vi "Finalize.vi"(3 "erreur in":errorcluster caption="eerror in", 5 "ref in":refnum<k7>) -> (0 "error out":errorcluster)   [LabVIEW 2010]
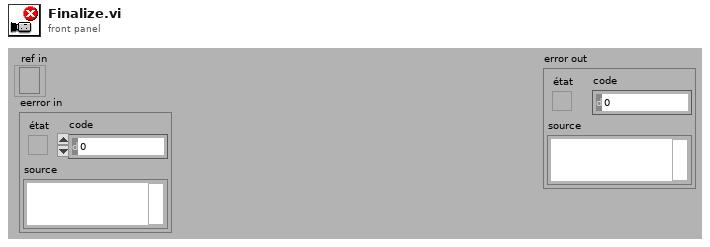
[diagram p1: front panel]
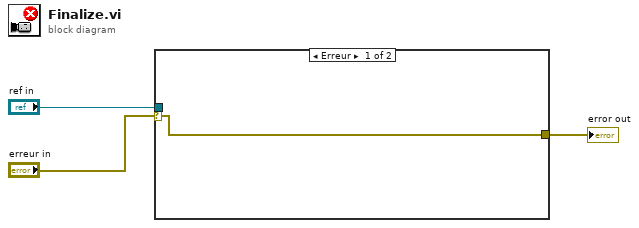
[diagram p0: block diagram]
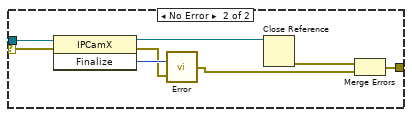
[diagram p2: hidden frame]
diagram:
  n1 = case shown="Erreur" "erreur in" {
    selector: "erreur in" -> [w4 w9]
    tunnel: "ref in" -> [_ w10]
    tunnel: [w4 w5] -> w1
    frame Error {
    }
    frame No Error {
      n2 = invoke class="IPCamX" method="Finalize"(reference=w10, error in=w9) -> (reference out=w11:refnum<k7>, error out=w7:errorcluster, "Finalize"=w8:i32)  [unwired: 1 in]
      n3 = call "Error.vi"("error in"=w7, "code"=w8) -> ("error out"=w6:errorcluster)
      n4 = Close Reference(reference=w11) -> (error out=w12:errorcluster)  [unwired: 1 in]
      n5 = Merge Errors(w12, w6) -> (w5:errorcluster)
    }
  }
  "error out" <- w1
